vi "多参数电源命令.vi"(10 "通电/断电":bool, 11 "队列":refnum<queue>) -> (3 "队列输出":refnum<queue>)   [LabVIEW 2016, in "PLC.lvlib"]
uses:
  PLC.lvlib
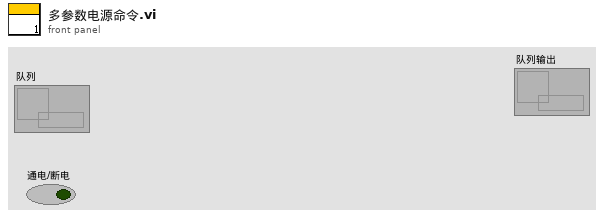
[diagram p1: front panel]
types:
  T1 = cluster{"命令":string, "数据":cluster{"starting address":u16, "holding register value":u16}}
  T2 = cluster{"命令":string, "data":cluster{"starting address":u16, "coil values":bool[]}}
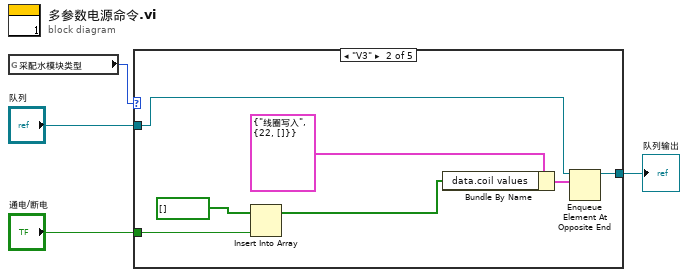
[diagram p0: block diagram]
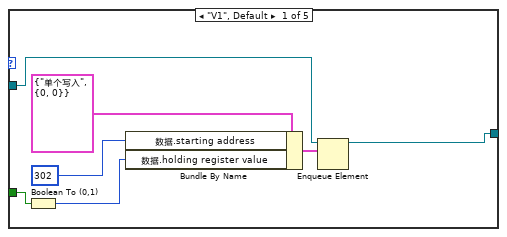
[diagram p2: hidden frame]
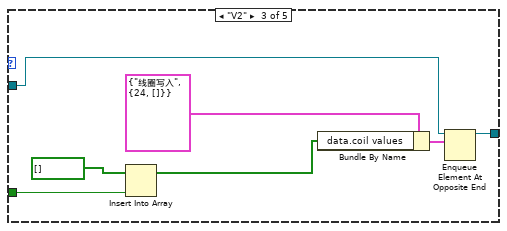
[diagram p3: hidden frame]
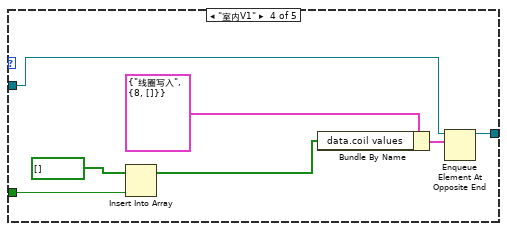
[diagram p4: hidden frame]
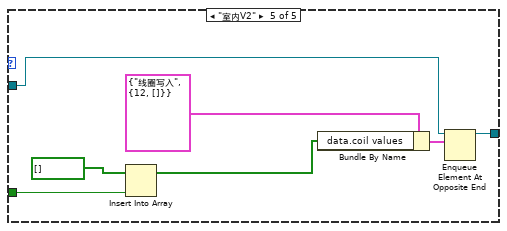
[diagram p5: hidden frame]
diagram:
  n1 = global read "系统设置全局变量.vi" "采配水模块类型"() -> (w1:enum16{"V1", "V2", "V3", "V4", "室内V1", "室内V2"})
  n2 = case shown="\"V3\"" w1 {
    tunnel: "队列" -> [w9 w17 w24 w31 w38]
    tunnel: [w8 w16 w23 w30 w37] -> w3
    tunnel: "通电/断电" -> [w6 w15 w22 w29 w36]
    frame "V1", Default {
      n3 = Boolean To (0,1)(Boolean=w6) -> (0, 1=w5:i16)
      n4 = Bundle By Name(cluster=T1 {"命令"="单个写入", "数据"={"starting address"=0, "holding register value"=0}} ("元素"), "数据.starting address"=u16 302, "数据.holding register value"=w5) -> (w7:T1)
      n5 = Enqueue Element(queue=w9, element=w7) -> (queue out=w8:refnum<queue>)  [unwired: 2 in, 2 out]
    }
    frame "V3" {
      n6 = Insert Into Array(array=bool[] [] ("data.coil values"), new element=w15) -> (w12:bool[])  [unwired: 1 in]
      n7 = Bundle By Name(cluster=T2 {"命令"="线圈写入", "data"={"starting address"=22, "coil values"=[]}} ("元素"), "data.coil values"=w12) -> (w18:T2)
      n8 = Enqueue Element At Opposite End(queue=w17, element=w18) -> (queue out=w16:refnum<queue>)  [unwired: 2 in, 2 out]
    }
    frame "V2" {
      n9 = Insert Into Array(array=bool[] [] ("data.coil values"), new element=w22) -> (w19:bool[])  [unwired: 1 in]
      n10 = Bundle By Name(cluster=T2 {"命令"="线圈写入", "data"={"starting address"=24, "coil values"=[]}} ("元素"), "data.coil values"=w19) -> (w25:T2)
      n11 = Enqueue Element At Opposite End(queue=w24, element=w25) -> (queue out=w23:refnum<queue>)  [unwired: 2 in, 2 out]
    }
    frame "室内V1" {
      n12 = Insert Into Array(array=bool[] [] ("data.coil values"), new element=w29) -> (w26:bool[])  [unwired: 1 in]
      n13 = Bundle By Name(cluster=T2 {"命令"="线圈写入", "data"={"starting address"=8, "coil values"=[]}} ("元素"), "data.coil values"=w26) -> (w32:T2)
      n14 = Enqueue Element At Opposite End(queue=w31, element=w32) -> (queue out=w30:refnum<queue>)  [unwired: 2 in, 2 out]
    }
    frame "室内V2" {
      n15 = Insert Into Array(array=bool[] [] ("data.coil values"), new element=w36) -> (w33:bool[])  [unwired: 1 in]
      n16 = Bundle By Name(cluster=T2 {"命令"="线圈写入", "data"={"starting address"=12, "coil values"=[]}} ("元素"), "data.coil values"=w33) -> (w39:T2)
      n17 = Enqueue Element At Opposite End(queue=w38, element=w39) -> (queue out=w37:refnum<queue>)  [unwired: 2 in, 2 out]
    }
  }
  "队列输出" <- w3
